vi "Extract String.vi"(8 "Resolution":string[][](array[string]), 11 "Condition":string[][](array[string])) -> (0 "배열 1":string[](array[string]) caption="표시형식, 최소눈금", 3 "배열 2":string[](array[string]) caption="최대, 최소, 단위", 5 "측정범위":dbl[](array[numeric]))   [LabVIEW 2020]
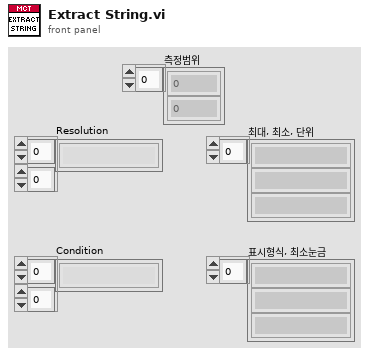
[diagram p1: front panel]
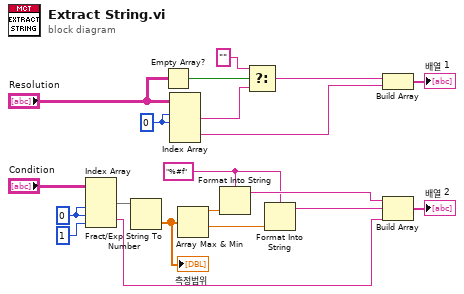
[diagram p0: block diagram]
diagram:
  w8 = 0 ("인덱스 (행)")
  w9 = "%#f" ("포맷 문자열")
  w17 = 0 ("인덱스 (행)")
  n1 = Index Array(array="Condition", index (col) #1=w17, index (row) #2=w17, index (col) #2=1 ("비활성화된 인덱스 (열)")) -> (element #1=w13:string[], element #2=w19:string)  [unwired: 1 in]
  n2 = Fract/Exp String To Number(string=w13) -> (number=w12:dbl[])  [unwired: 3 in, 1 out]
  "측정범위" <- w12
  n3 = Empty Array?(array="Resolution") -> (empty?=w5:bool)
  n4 = Index Array(array="Resolution", index (row) #1=w8, index (col) #1=w8) -> (element #1=w3:string, element #2=w1:string)  [unwired: 2 in]
  n5 = Array Max & Min(array=w12) -> (max value=w11:dbl, min value=w10:dbl)  [unwired: 2 out]
  n6 = Format Into String(format string=w9, w11) -> (resulting string=w15:string)  [unwired: 2 in, 1 out]
  n7 = Select(t="" ("원소"), s=w5, f=w3) -> (s? t:f=w2:string)
  n8 = Format Into String(format string=w9, w10) -> (resulting string=w16:string)  [unwired: 2 in, 1 out]
  n9 = Build Array(w2, w1) -> (→"배열 1":string[])
  n10 = Build Array(w15, w16, w19) -> (→"배열 2":string[])
